vi "Path From Parameter.vi"(10 "Path Parameter":string, 11 "Working Directory":path) -> (2 "Full Path":path)   [LabVIEW 2015, in "CLI.lvclass"]
doc: "Takes the current working directory and any input arguments which represents paths and converts them to an absolute path.\n\nIf they already are an absolute path they are ignored."
uses:
  CLI.lvclass
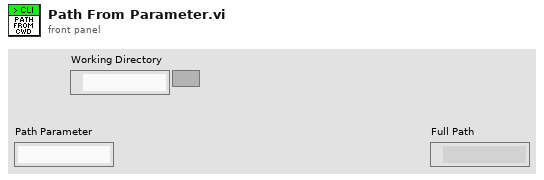
[diagram p1: front panel]
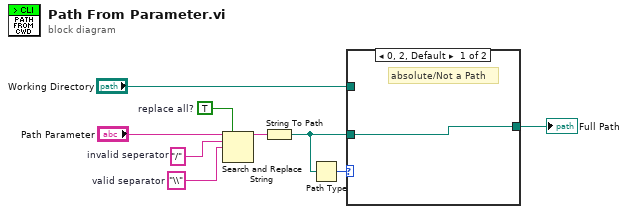
[diagram p0: block diagram]
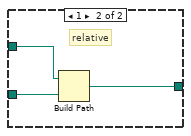
[diagram p2: hidden frame]
diagram:
  w1 = TRUE  # replace all?
  w2 = "\\"  # valid separator
  w3 = "/"  # invalid seperator
  n1 = Search and Replace String(replace all?=w1, input string="Path Parameter", search string=w3, replace string=w2) -> (result string=w4:string)  [unwired: 4 in, 3 out]
  n2 = String To Path(string=w4) -> (path=w7:path)
  n3 = Path Type(1:w7) -> (0:w6:i16)
  n4 = case shown="0, 2, Default" w6 {
    tunnel: "Working Directory" -> [_ w13]
    tunnel: [w10 w12] -> w8
    tunnel: w7 -> [w10 w11]
    frame 0, 2, Default {
      # "absolute/Not a Path"
    }
    frame 1 {
      # "relative"
      n5 = Build Path(base path=w13, name or relative path=w11) -> (appended path=w12:path)
    }
  }
  "Full Path" <- w8
